vi "ImageFile_GetFolderImageAndRotate.vi"(8 "error in (no error)":errorcluster, 11 "Folder Image Files":refnum<vi>) -> (0 "error out":errorcluster, 3 "File Path":path)   [LabVIEW 2019]
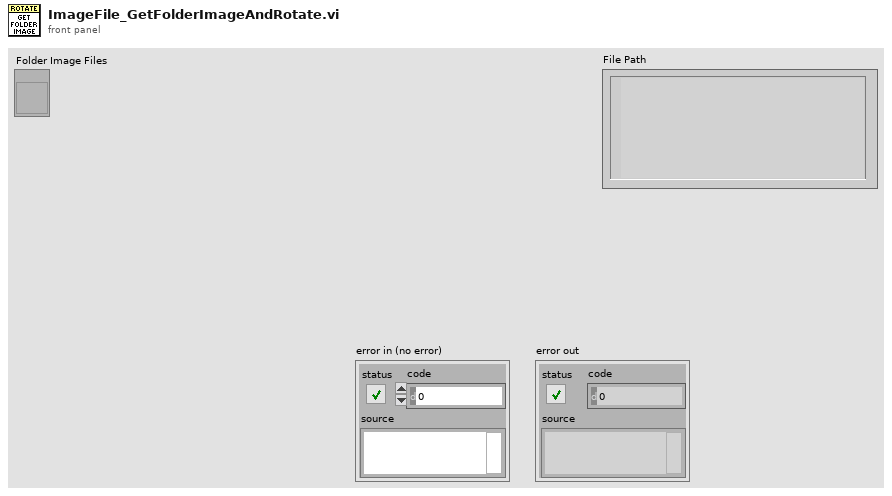
[diagram p1: front panel]
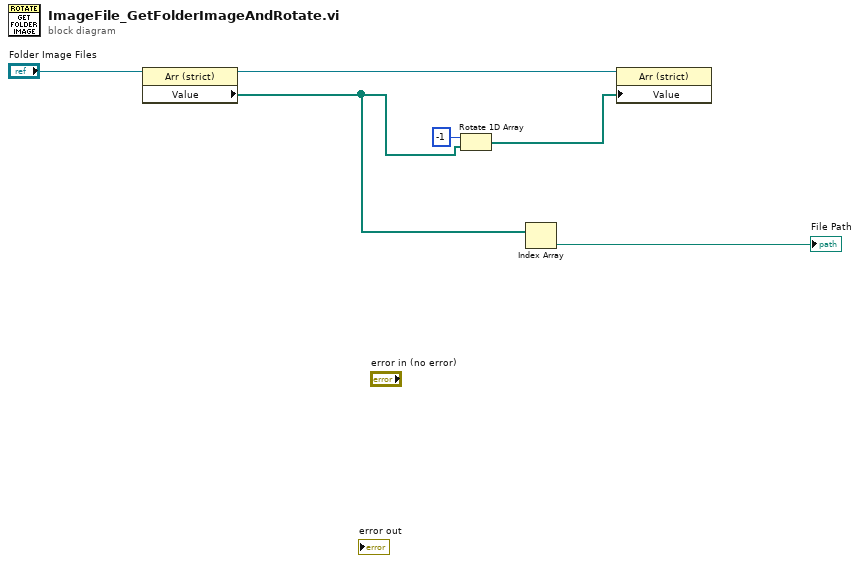
[diagram p0: block diagram]
diagram:
  n1 = property class="Arr (strict)"(reference="Folder Image Files") -> (reference out=w4:refnum<vi>, "Value"=w2:path[])  [unwired: 1 in, 1 out]
  n2 = Rotate 1D Array(1:w2, 2:-1 ("n")) -> (0:w1:path[])
  n3 = Index Array(array=w2) -> (element=→"File Path":path)  [unwired: 1 in]
  n4 = property class="Arr (strict)"(reference=w4, "Value"=w1) -> ()  [unwired: 1 in, 2 out]
